vi "DriveNetwork.vi"(8 "error in (no error)":errorcluster) -> (0 "error out":errorcluster)   [LabVIEW 2020]
doc: "Network for Drive\n\nInputs:\n -- Error in -- Error cluster -- propagated error input\n\nOutputs:\n -- Error out -- Error cluster -- progated error output"
uses:
  DriveGlobal.vi
  <vilib>/Rock Robotics/Network Tables/NT Write Number.vi
  <vilib>/Rock Robotics/Network Tables/NT Write Boolean.vi
  <vilib>/Rock Robotics/Network Tables/NT Read Boolean.vi
  <vilib>/Rock Robotics/WPI/ThirdParty/JAS_Junk/TrajLib/Trajectory_Library.lvlib
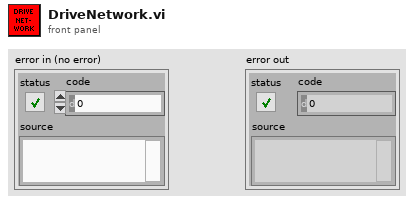
[diagram p1: front panel]
types:
  T1 = enum16{"Moving Average", "Low Pass 1st Order Butterworth", "Low Pass 2nd Order Butterworth", "High Pass 1st Order Butterworth", "High Pass 2nd Order Butterworth"}
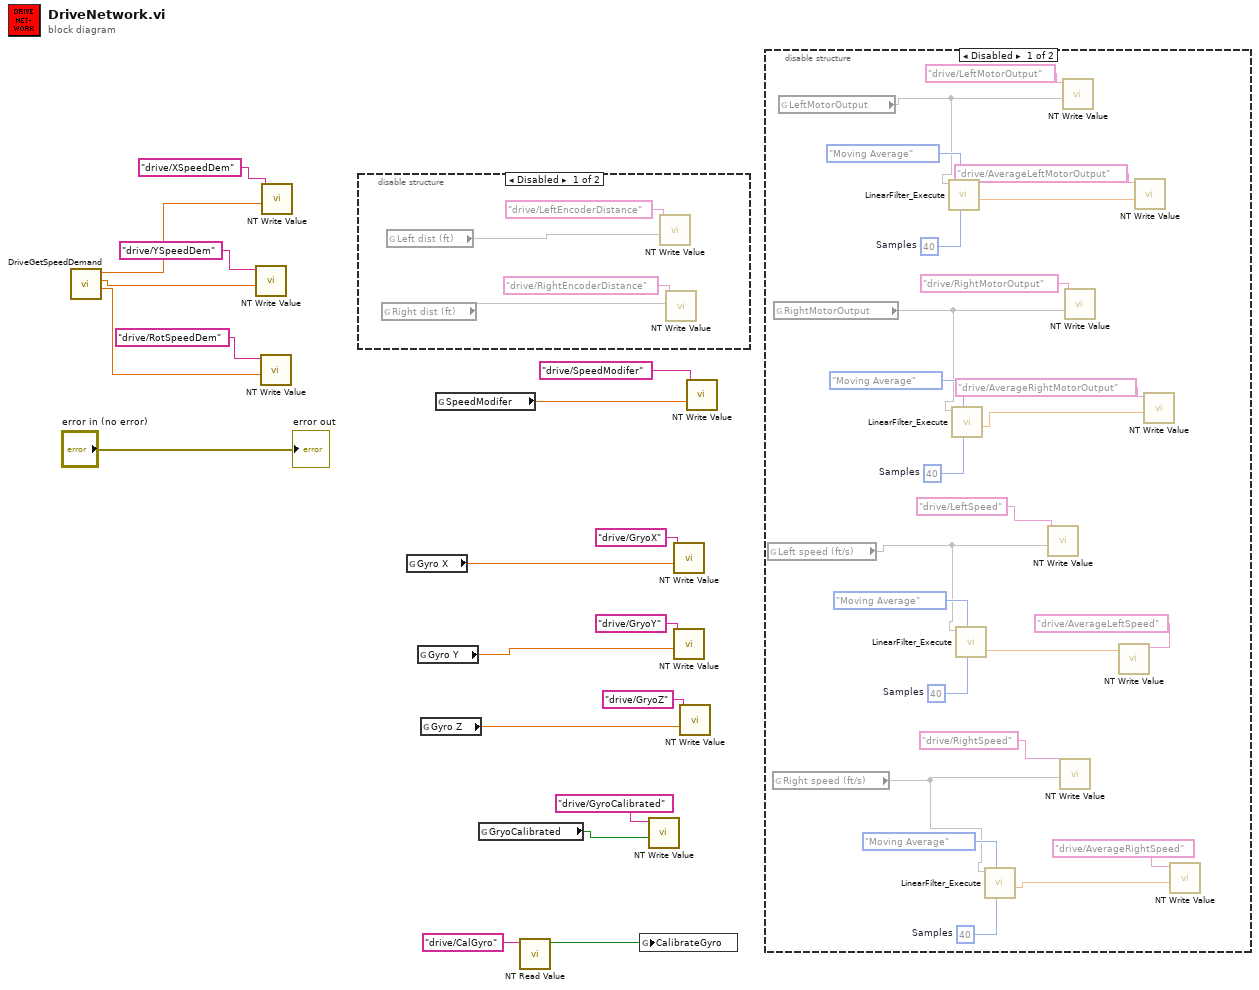
[diagram p0: block diagram]
diagram:
  n1 = call "DriveGetSpeedDemand.vi"() -> ("vOmega"=w1:dbl, "vY"=w17:dbl, "vX"=w18:dbl)  [unwired: 8 in, 1 out]
  n2 = call-poly <vilib>:"NT Write Value.vi"("value"=w17, "name"="drive/YSpeedDem") -> ()  [unwired: 9 in, 1 out]
  n3 = call-poly <vilib>:"NT Write Value.vi"("value"=w1, "name"="drive/RotSpeedDem") -> ()  [unwired: 9 in, 1 out]
  n4 = call-poly <vilib>:"NT Write Value.vi"("value"=w18, "name"="drive/XSpeedDem") -> ()  [unwired: 9 in, 1 out]
  n5 = disable-structure shown="Disabled" {
    frame Disabled {
      n6 = global read "DriveGlobal.vi" "Right dist (ft)"() -> (w21)
      n7 = global read "DriveGlobal.vi" "Left dist (ft)"() -> (w20)
      n8 = call-poly <vilib>:"NT Write Value.vi"("value"=w20, "name"="drive/LeftEncoderDistance") -> ()  [unwired: 9 in, 1 out]
      n9 = call-poly <vilib>:"NT Write Value.vi"("value"=w21, "name"="drive/RightEncoderDistance") -> ()  [unwired: 9 in, 1 out]
    }
    frame Enabled {
    }
  }
  n10 = global read "DriveGlobal.vi" "Gyro X"() -> (w11:dbl)
  n11 = global read "DriveGlobal.vi" "Gyro Y"() -> (w12:dbl)
  n12 = global read "DriveGlobal.vi" "Gyro Z"() -> (w13:dbl)
  n13 = global read "DriveGlobal.vi" "SpeedModifer"() -> (w9:dbl)
  n14 = global read "DriveGlobal.vi" "GryoCalibrated"() -> (w3:bool)
  n15 = call-poly <vilib>:"NT Read Value.vi"("name"="drive/CalGyro") -> ("value"=w4:bool)  [unwired: 8 in, 2 out]
  n16 = global write "DriveGlobal.vi" "CalibrateGyro"(w4) -> ()
  n17 = call-poly <vilib>:"NT Write Value.vi"("value"=w3, "name"="drive/GyroCalibrated") -> ()  [unwired: 9 in, 1 out]
  n18 = call-poly <vilib>:"NT Write Value.vi"("value"=w11, "name"="drive/GryoX") -> ()  [unwired: 9 in, 1 out]
  n19 = call-poly <vilib>:"NT Write Value.vi"("value"=w12, "name"="drive/GryoY") -> ()  [unwired: 9 in, 1 out]
  n20 = call-poly <vilib>:"NT Write Value.vi"("value"=w13, "name"="drive/GryoZ") -> ()  [unwired: 9 in, 1 out]
  n21 = call-poly <vilib>:"NT Write Value.vi"("value"=w9, "name"="drive/SpeedModifer") -> ()  [unwired: 9 in, 1 out]
  n22 = disable-structure shown="Disabled" {
    frame Disabled {
      w39 = 40  # Samples
      w41 = 40  # Samples
      w43 = 40  # Samples
      w45 = 40  # Samples
      n23 = global read "DriveGlobal.vi" "Left speed (ft/s)"() -> (w32)
      n24 = global read "DriveGlobal.vi" "Right speed (ft/s)"() -> (w33)
      n25 = global read "DriveGlobal.vi" "RightMotorOutput"() -> (w31)
      n26 = global read "DriveGlobal.vi" "LeftMotorOutput"() -> (w30)
      n27 = call <vilib>:"LinearFilter_Execute.vi"("Samples"=w39, "Filter Type"=T1."Moving Average", "Input"=w30) -> ("Output"=w29:dbl)  [unwired: 7 in, 1 out]
      n28 = call <vilib>:"LinearFilter_Execute.vi"("Samples"=w41, "Filter Type"=T1."Moving Average", "Input"=w31) -> ("Output"=w28:dbl)  [unwired: 7 in, 1 out]
      n29 = call <vilib>:"LinearFilter_Execute.vi"("Samples"=w43, "Filter Type"=T1."Moving Average", "Input"=w32) -> ("Output"=w27:dbl)  [unwired: 7 in, 1 out]
      n30 = call <vilib>:"LinearFilter_Execute.vi"("Samples"=w45, "Filter Type"=T1."Moving Average", "Input"=w33) -> ("Output"=w26:dbl)  [unwired: 7 in, 1 out]
      n31 = call-poly <vilib>:"NT Write Value.vi"("value"=w32, "name"="drive/LeftSpeed") -> ()  [unwired: 9 in, 1 out]
      n32 = call-poly <vilib>:"NT Write Value.vi"("value"=w33, "name"="drive/RightSpeed") -> ()  [unwired: 9 in, 1 out]
      n33 = call-poly <vilib>:"NT Write Value.vi"("value"=w30, "name"="drive/LeftMotorOutput") -> ()  [unwired: 9 in, 1 out]
      n34 = call-poly <vilib>:"NT Write Value.vi"("value"=w31, "name"="drive/RightMotorOutput") -> ()  [unwired: 9 in, 1 out]
      n35 = call-poly <vilib>:"NT Write Value.vi"("value"=w27, "name"="drive/AverageLeftSpeed") -> ()  [unwired: 9 in, 1 out]
      n36 = call-poly <vilib>:"NT Write Value.vi"("value"=w29, "name"="drive/AverageLeftMotorOutput") -> ()  [unwired: 9 in, 1 out]
      n37 = call-poly <vilib>:"NT Write Value.vi"("value"=w28, "name"="drive/AverageRightMotorOutput") -> ()  [unwired: 9 in, 1 out]
      n38 = call-poly <vilib>:"NT Write Value.vi"("value"=w26, "name"="drive/AverageRightSpeed") -> ()  [unwired: 9 in, 1 out]
    }
    frame Enabled {
    }
  }
  "error out" <- "error in (no error)"
